vi "Output 信息检测.vi"(9 "Output配置信息":string[][](table)=[["名称", "点位", "索引号"], ["三色灯红", "Y100", "0"], ["三色灯绿", "Y101", "1"], ["三色灯黄", "Y102", "2"], ["蜂鸣器", "Y103", "3"], ["上层真空电磁阀", "Y104", "4"], ["下层真空电磁阀", "Y105", "5"], ["传送抓手气缸", "Y106", "6"], ["上层产品定位气缸", "Y107", "7"], ["下层产品定位气缸", "Y110", "8"], ["起子1吸附真空", "Y111", "9"], ["起子2吸附真空", "Y112", "10"], ["起子3吸附真空", "Y113", "11"], ["起子4吸附真空", "Y114", "12"], ["起子1吹气电磁阀", "Y115", "13"], ["起子2吹气电磁阀", "Y116", "14"], ["起子3吹气电磁阀", "Y117", "15"], ["起子4吹气电磁阀", "Y120", "16"], ["光源", "Y121", "17"], ["Feed1指示灯", "Y122", "18"], ["Feed2指示灯", "Y123", "19"], ["Feed3指示灯", "Y124", "20"], ["Feed4指示灯", "Y125", "21"], ["上站取料完成反馈", "Y126", "22"], ["下站投料完成反馈", "Y127", "23"], ["上站给出请求信号", "Y130", "24"], ["下站给出答复信号", "Y131", "25"]], 11 "输出":T1) -> (2 "Output Error":string[](array[string]))   [LabVIEW 2017]
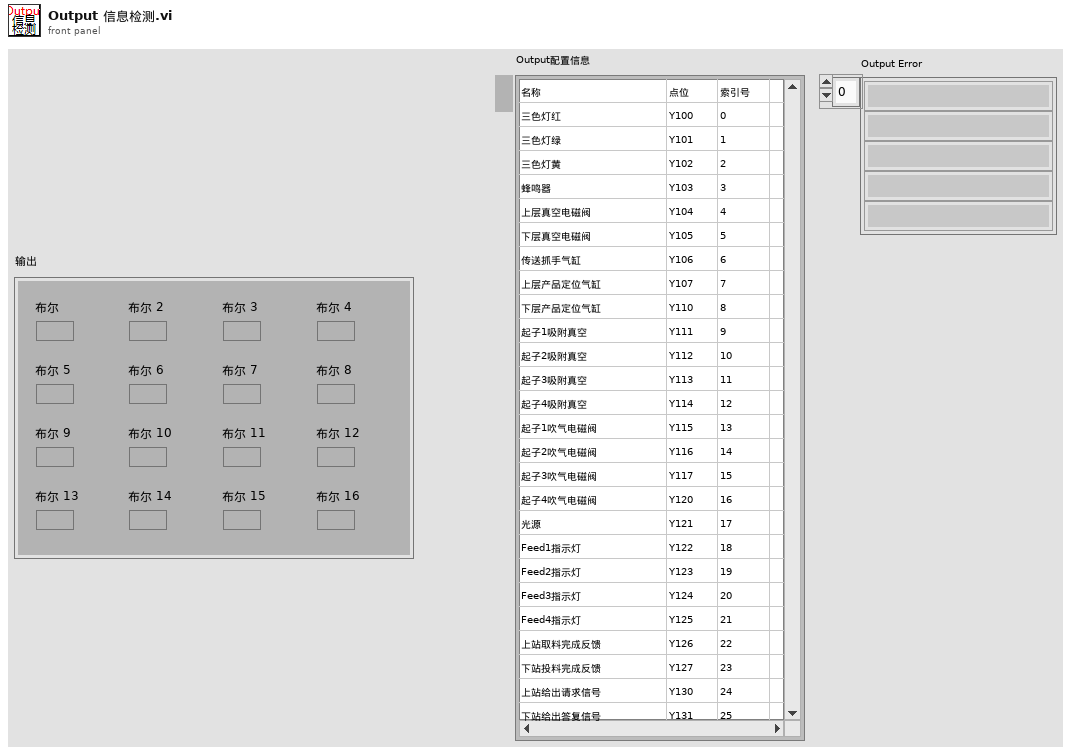
[diagram p1: front panel]
types:
  T1 = typedef "output控件.ctl" = cluster{"布尔":bool, "布尔 2":bool, "布尔 3":bool, "布尔 4":bool, "布尔 5":bool, "布尔 6":bool, "布尔 7":bool, "布尔 8":bool, "布尔 9":bool, "布尔 10":bool, "布尔 11":bool, "布尔 12":bool, "布尔 13":bool, "布尔 14":bool, "布尔 15":bool, "布尔 16":bool}
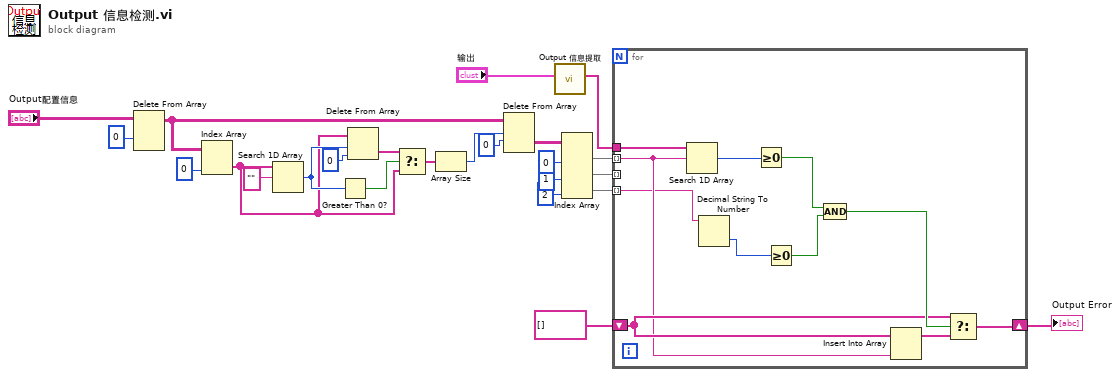
[diagram p0: block diagram]
diagram:
  n1 = Delete From Array(array="Output配置信息", index (row)=0 ("索引 (行)")) -> (array with subset deleted=w12:string[][])  [unwired: 2 in, 1 out]
  n2 = Index Array(array=w12, index (col)=0 ("禁用的索引 (列)")) -> (element=w15:string[])  [unwired: 1 in]
  n3 = Search 1D Array(1D array=w15, element="") -> (index of element=w19:i32)  [unwired: 1 in]
  n4 = Greater Than 0?(x=w19) -> (x > 0?=w20:bool)
  n5 = Delete From Array(array=w15, length=w19, index=0 ("索引")) -> (deleted portion=w17:string[])  [unwired: 1 out]
  n6 = Select(t=w17, s=w20, f=w15) -> (s? t:f=w14:string[])
  n7 = Array Size(array=w14) -> (size(s)=w16:i32)
  n8 = Delete From Array(array=w12, length=w16, index (row)=0 ("索引 (行)")) -> (deleted portion=w1:string[][])  [unwired: 1 in, 1 out]
  n9 = call "Output 信息提取.vi"("输出"="输出") -> ("Output 信息配置"=w3:string[])  [unwired: 10 in]
  n10 = Index Array(array=w1, index (col) #1=0 ("禁用的索引 (列)"), index (col) #2=1 ("禁用的索引 (列)"), index (col) #3=2 ("禁用的索引 (列)")) -> (element #1=w7:string[], element #2=w6:string[], element #3=w5:string[])  [unwired: 3 in]
  n11 = for {
    tunnel: w7 -> [w28] mode=indexing
    tunnel: w6 -> [_] mode=indexing
    tunnel: w5 -> [w27] mode=indexing
    shift-right: [w30] -> w2
    shift-left: string[] [] -> [w32]
    tunnel: w3 -> [w29]
    n12 = Search 1D Array(1D array=w29, element=w28) -> (index of element=w35:i32)  [unwired: 1 in]
    n13 = Decimal String To Number(string=w27) -> (number=w26:i32)  [unwired: 2 in, 1 out]
    n14 = Greater Or Equal To 0?(x=w35) -> (x >= 0?=w34:bool)
    n15 = Greater Or Equal To 0?(x=w26) -> (x >= 0?=w25:bool)
    n16 = Compound Arithmetic op=AND(w34, w25) -> (w33:bool)
    n17 = Insert Into Array(array=w32, new element=w28) -> (w31:string[])  [unwired: 1 in]
    n18 = Select(t=w32, s=w33, f=w31) -> (s? t:f=w30:string[])
  }
  "Output Error" <- w2
